vi "ma_run.vi"() -> ()   [LabVIEW 2013]
panel:
  out "x1":dbl
  out "x2":dbl
  out "x3":dbl
  out "最終堆疊版 2":bool[][](array[boolean])
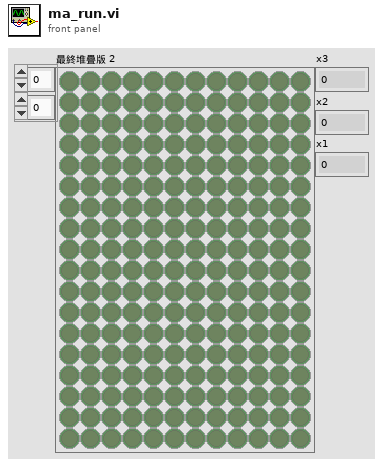
[diagram p1: front panel]
types:
  T1 = typedef "KNR3 Reference.ctl" = cluster{"FPGA Session":refnum<class "FPGA Interface Base.lvclass">, "Resource":T2}
  T2 = typedef "Resource.ctl" = enum16{"KNRm_DDRC", "KNRm_DDDD", "KNRm_DDDR", "KNRm_DDDC", "KNR"}
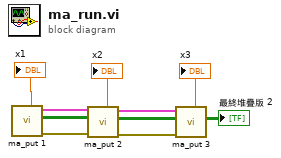
[diagram p0: block diagram]
diagram:
  n1 = call "ma_put 1.vi"() -> ("error out 4"=w6:errorcluster, "最終堆疊版"=w8:bool[][], "KNR out"=w10:T1, "x1"=→"x1":dbl)  [unwired: 8 in]
  n2 = call "ma_put 2.vi"("Error"=w6, "初始進入"=w8, "KNR in"=w10) -> ("error out 4"=w5:errorcluster, "最終堆疊版 2"=w7:bool[][], "KNR out"=w9:T1, "x2"=→"x2":dbl)  [unwired: 5 in]
  n3 = call "ma_put 3.vi"("Error"=w5, "初始進入"=w7, "KNR in"=w9) -> ("最終堆疊版 2"=→"最終堆疊版 2":bool[][], "x3"=→"x3":dbl)  [unwired: 5 in, 2 out]
